vi "MakeDataFileNames.vi"(0 "Root Data Folder":path=path "C:/Data", 1 "File format":T1, 3 "Include time":bool, 5 "Index digits":i32=3, 7 "Index file":string="index.txt", 9 "Interactive":bool=TRUE, 11 "Error In":errorcluster, 12 "File Prefix":string="ms", 13 "File middle":string="ms", 14 "Time Stamp (default 0 = now)":timestamp) -> (4 "Data File  Path":path, 6 "Settings File Path":path, 8 "Try count":i32, 10 "Index  File Path":path, 15 "Error Out":errorcluster)   [LabVIEW 2024]
uses:
  Controls/File formats.ctl
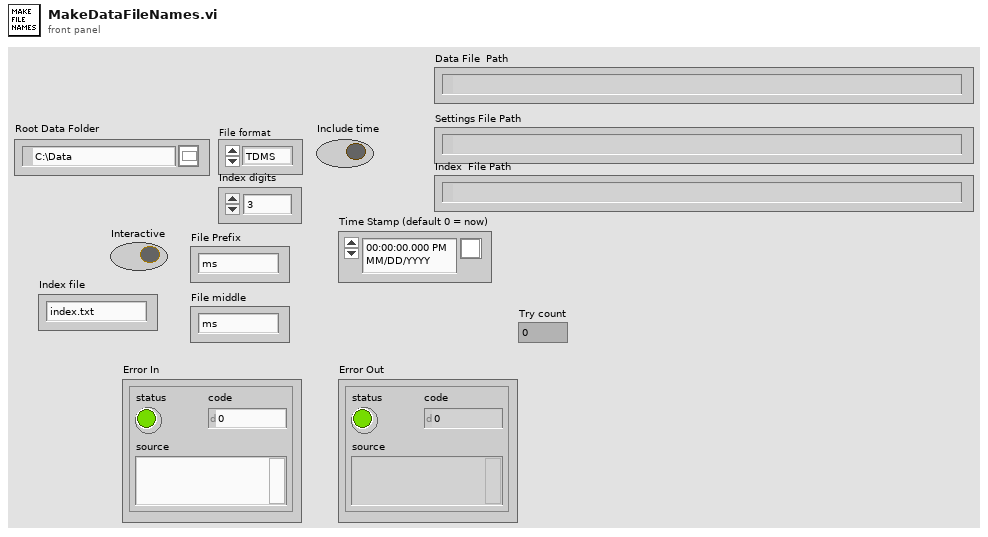
[diagram p1: front panel]
types:
  T1 = typedef "File formats.ctl" = enum16{"TDMS", "ASCII", "BINARY"}
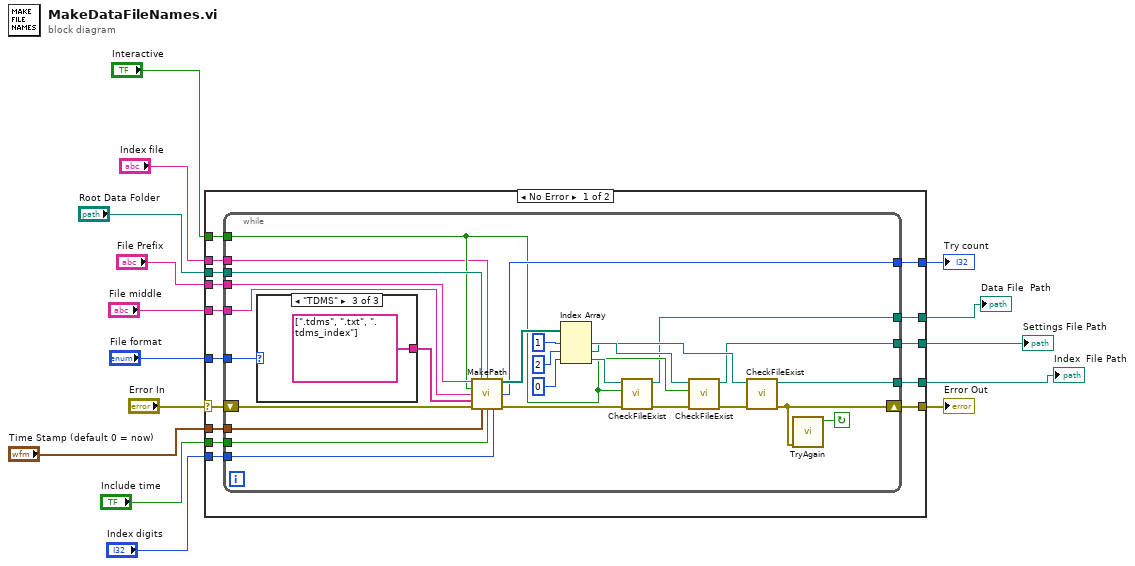
[diagram p0: block diagram]
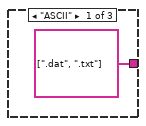
[diagram p2: hidden frame]
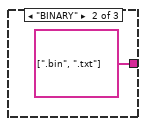
[diagram p3: hidden frame]
diagram:
  n1 = case shown="No Error" "Error In" {
    selector: "Error In" -> [w19 w61]
    tunnel: [w30 w61] -> w15
    tunnel: "Root Data Folder" -> [w29 _]
    tunnel: "Index digits" -> [w28 _]
    tunnel: "Time Stamp (default 0 = now)" -> [w27 _]
    tunnel: "File Prefix" -> [w26 _]
    tunnel: "File middle" -> [w25 _]
    tunnel: [w24 _] -> w9
    tunnel: "Include time" -> [w23 _]
    tunnel: "Interactive" -> [w22 _]
    tunnel: "Index file" -> [w21 _]
    tunnel: "File format" -> [w20 _]
    tunnel: [w18 _] -> w3
    tunnel: [w17 _] -> w2
    tunnel: [w16 _] -> w1
    frame No Error {
      n2 = while {
        shift-right: [w48] -> w30
        shift-left: w19 -> [w50]
        tunnel: w29 -> [w43]
        tunnel: w28 -> [w42]
        tunnel: w27 -> [w41]
        tunnel: w26 -> [w40]
        tunnel: w25 -> [w39]
        tunnel: [w38] -> w24
        tunnel: w23 -> [w37]
        tunnel: w22 -> [w36]
        tunnel: w21 -> [w35]
        tunnel: w20 -> [w34]
        tunnel: [w33] -> w18
        tunnel: [w32] -> w17
        tunnel: [w31] -> w16
        stop <- w57 continue-if-true
        n3 = case shown="\"TDMS\"" w34 {
          tunnel: [string[] [".dat", ".txt"] string[] [".bin", ".txt"] string[] [".tdms", ".txt", ".tdms_index"]] -> w54
          frame "ASCII" {
          }
          frame "BINARY" {
          }
          frame "TDMS" {
          }
        }
        n4 = call "MakePath.vi"("File Prefix"=w40, "Root Data Folder"=w43, "Index file"=w35, "Interactive"=w36, "File middle"=w39, "Extentions"=w54, "Error In"=w50, "Time Stamp (default 0 = now)"=w41, "Include time"=w37, "Index digits"=w42) -> ("Paths out"=w51:path[], "Try count"=w38:i32, "Error Out"=w56:errorcluster)  [unwired: 2 in, 1 out]
        n5 = Index Array(array=w51, index #1=1 ("index"), index #2=2 ("index"), index #3=0 ("index")) -> (element #1=w52:path, element #2=w46:path, element #3=w44:path)
        n6 = call "CheckFileExist.vi"("error in (no error) 2"=w56, "Interactive"=w36, "File Path"=w44) -> ("error out"=w55:errorcluster, "File out"=w33:path)  [unwired: 7 out]
        n7 = call "CheckFileExist.vi"("error in (no error) 2"=w55, "Interactive"=w36, "File Path"=w52) -> ("error out"=w49:errorcluster, "File out"=w32:path)  [unwired: 1 in, 6 out]
        n8 = call "CheckFileExist.vi"("error in (no error) 2"=w49, "File Path"=w46) -> ("error out"=w48:errorcluster, "File out"=w31:path)  [unwired: 2 in, 6 out]
        n9 = call "TryAgain.vi"("error in (no error)"=w48) -> ("Try again"=w57:bool)  [unwired: 6 out]
      }
    }
    frame Error {
    }
  }
  "Error Out" <- w15
  "Try count" <- w9
  "Data File  Path" <- w3
  "Settings File Path" <- w2
  "Index  File Path" <- w1
